vi "RemovePeaks1.vi"(11 "wfm in":waveform(dbl)) -> (2 "original + denoised":waveform(dbl)[](graph), 3 "denoised wfm":waveform(dbl)(graph))   [LabVIEW 2025]
uses:
  <vilib>/gmath/statdist.llb/st_Percentiles (scalar).vi
  <vilib>/gmath/NI_Gmath.lvlib
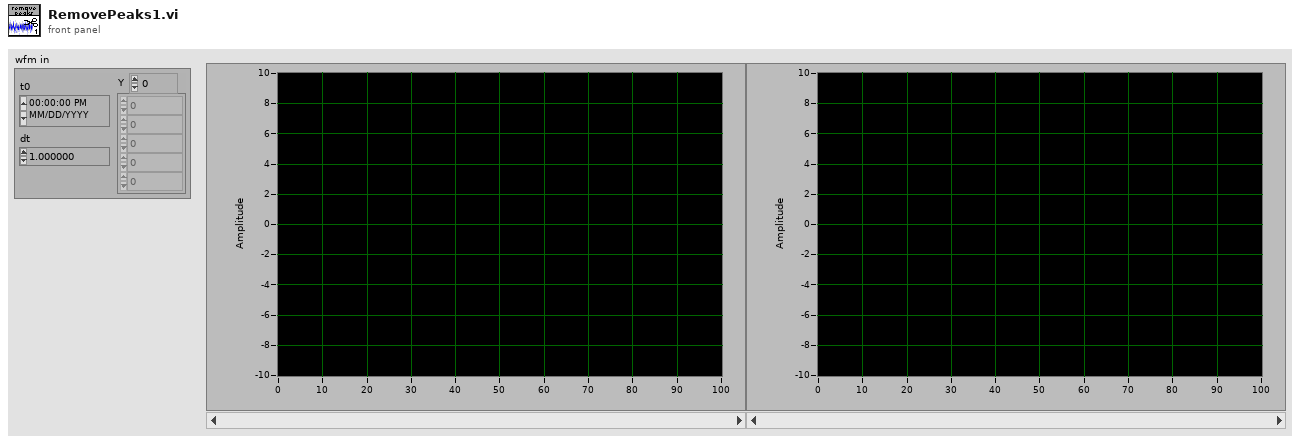
[diagram p1: front panel]
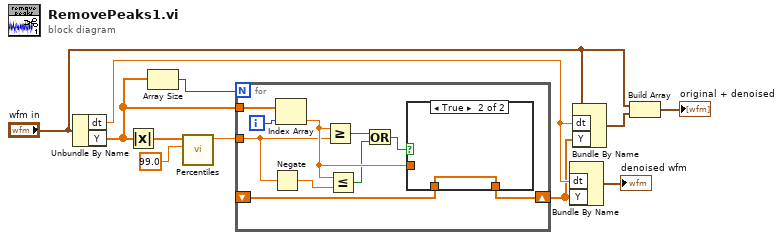
[diagram p0: block diagram]
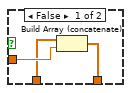
[diagram p2: hidden frame]
diagram:
  n1 = Unbundle By Name("wfm in") -> ("dt"=w5:dbl, "Y"=w8:dbl[])
  n2 = Absolute Value(x=w8) -> (abs(x)=w10:dbl[])
  n3 = Array Size(array=w8) -> (size(s)=w9:i32)
  n4 = call-poly <vilib>:"Percentiles.vi"("p"=99.0, "x array"=w10) -> ("percentile"=w7:dbl)  [unwired: 8 in, 1 out]
  n5 = for {
    N: w9 -> [_]
    tunnel: w8 -> [w20]
    tunnel: w7 -> [w15]
    shift-right: [w19] -> w4
    shift-left: _ -> [w18]
    i -> [w21]
    n6 = Negate(x=w15) -> (-x=w16:dbl)
    n7 = Index Array(array=w20, index=w21) -> (element=w17:dbl)
    n8 = Greater Or Equal?(x=w17, y=w15) -> (x >= y?=w14:bool)
    n9 = Less Or Equal?(x=w17, y=w16) -> (x <= y?=w13:bool)
    n10 = Or(x=w14, y=w13) -> (x .or. y?=w12:bool)
    n11 = case shown="True" w12 {
      tunnel: w17 -> [w23 _]
      tunnel: [w24 w25] -> w19
      tunnel: w18 -> [w22 w25]
      frame False {
        n12 = Build Array (concatenate)(w22, w23) -> (w24:dbl[])
      }
      frame True {
      }
    }
  }
  n13 = Bundle By Name("dt"=w5, "Y"=w4) -> (→"denoised wfm":waveform(dbl))  [unwired: 1 in]
  n14 = Bundle By Name(cluster="wfm in", "dt"=w5, "Y"=w4) -> (w2:waveform(dbl))
  n15 = Build Array("wfm in", w2) -> (→"original + denoised":waveform(dbl)[])
